vi "ttm_moveToSetpoint_poller.vi"   [LabVIEW 2011]
types:
  T1 = cluster{"Name":string, "Type":i32, "SI Full Scale":dbl, "Full Scale":dbl, "Units String":string, "Display Format":string, "Gauge Length":dbl}[][]
  T2 = cluster{"Device ID":i32, "Device Name":string, "Device Type":i32}[]
  T3 = cluster{"Double":dbl, "Double":dbl, "setpointTime":dbl, "setpointTime":dbl}
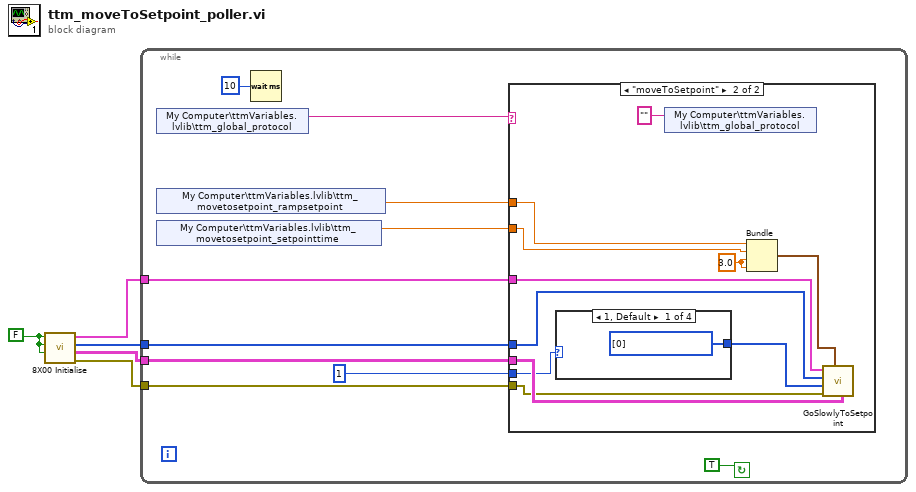
[diagram p0: block diagram]
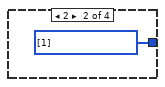
[diagram p3: hidden frame]
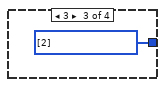
[diagram p4: hidden frame]
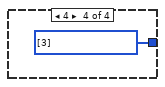
[diagram p5: hidden frame]
diagram:
  w1 = FALSE ("Create Console? (T)")
  n1 = call "8X00 Initialise.vi"("Reset?"=w1, "Create DVM? (T)"=w1, "Create Console? (T)"=w1) -> ("error out"=w2:errorcluster, "Channel Data"=w3:T1, "Axis Selector"=w4:i32[], "Axis Information"=w5:T2)  [unwired: 1 in]
  n2 = while {
    tunnel: w5 -> [w14]
    tunnel: w4 -> [w13]
    tunnel: w3 -> [w12]
    tunnel: w2 -> [w11]
    stop <- TRUE continue-if-true
    n3 = shared-variable "My Computer\\ttmVariables.lvlib\\ttm_global_protocol"() -> (w7:string)  [unwired: 1 in, 1 out]
    n4 = shared-variable "My Computer\\ttmVariables.lvlib\\ttm_movetosetpoint_rampsetpoint"() -> (w10:dbl)  [unwired: 1 in, 1 out]
    n5 = shared-variable "My Computer\\ttmVariables.lvlib\\ttm_movetosetpoint_setpointtime"() -> (w8:dbl)  [unwired: 1 in, 1 out]
    n6 = Wait (ms)(milliseconds to wait=u32 10) -> ()  [unwired: 1 out]
    n7 = case shown="\"moveToSetpoint\"" w7 {
      tunnel: w14 -> [_ w25]
      tunnel: w13 -> [_ w24]
      tunnel: w12 -> [_ w23]
      tunnel: w11 -> [_ w22]
      tunnel: w10 -> [_ w26]
      tunnel: 1 ("channelInt") -> [_ w19]
      tunnel: w8 -> [_ w18]
      frame "False", Default {
      }
      frame "moveToSetpoint" {
        w17 = 3.0 ("setpointTime")
        n8 = case shown="1, Default" w19 {
          tunnel: [w27 w28 w29 w30] -> w21
          frame 1, Default {
            w27 = u16[] [0] items=["Channel 1", "Channel 2", "Channel 3", "Channel 4"] ("Choose channel to apply\nthe setpoint")
          }
          frame 2 {
            w28 = u16[] [1] items=["Channel 1", "Channel 2", "Channel 3", "Channel 4"] ("Choose channel to apply\nthe setpoint")
          }
          frame 3 {
            w29 = u16[] [2] items=["Channel 1", "Channel 2", "Channel 3", "Channel 4"] ("Choose channel to apply\nthe setpoint")
          }
          frame 4 {
            w30 = u16[] [3] items=["Channel 1", "Channel 2", "Channel 3", "Channel 4"] ("Choose channel to apply\nthe setpoint")
          }
        }
        n9 = shared-variable "My Computer\\ttmVariables.lvlib\\ttm_global_protocol"("" ("protocol")) -> ()  [unwired: 1 in, 1 out]
        n10 = Bundle("Double"=w26, "Double"=w18, "setpointTime"=w17, "setpointTime"=w17) -> (w20:T3)  [unwired: 1 in]
        n11 = call "GoSlowlyToSetpoint.vi"("Channel Data"=w23, "Input cluster"=w20, "error in (no error)"=w22, "Channels"=w21, "Axis Selector"=w24, "Axis Information"=w25) -> ()  [unwired: 2 in, 4 out]
      }
    }
  }
